vi "FourierTransform.vi"(3 "Image In":T1 {"Dialogs" format="%.0b"}) -> (0 "Complex FT":cdb[][](array[numeric]) format="%.2f", 1 "Image Out":T1 {"Dialogs" format="%.0b"})   [LabVIEW 2024]
doc: "This VI calculates the DFT (or FFT) of the image and returns the 2D complex array and puts the magnitude (log scaled) in the image area. It only works on greyscale images."
uses:
  <userlib>/ImageProcessing/QTLIB_2595_LV86/QT_Image.ctl
panel:
  # "This VI calculates the DFT (or FFT) of the image and\nreturns the 2D complex array and puts the magnitude \n(log scaled) in the image area.  It only works on greyscale images."
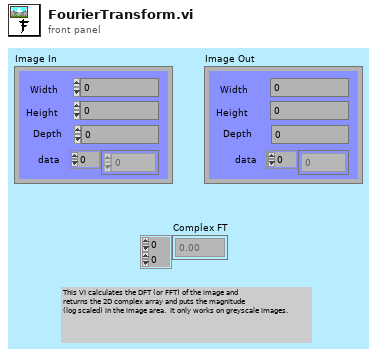
[diagram p1: front panel]
types:
  T1 = typedef "QT_Image.ctl" = cluster{"Width":i32, "Height":i32, "Depth":i32, "data":u8[], "Compressed data":u8[], "Color table":u32[], "Duration":i32, "Options":i32, "Timestamp":i32, "ID":i32, "Reserved":i32, "Dialogs":u32}
  T2 = enum16{"Same depth", "8 bit only", "1 image,8bit"}
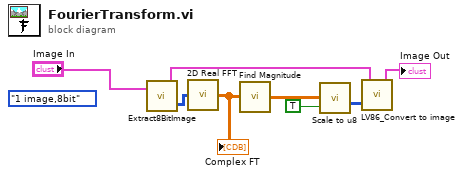
[diagram p0: block diagram]
diagram:
  (unwired) T2."1 image,8bit" ("Task")
  n1 = call <userlib>:"Extract8BitImage.vi"("Image in"="Image In") -> ("Intensity Graph"=w6:u8[][], "Image out"=w7:T1)  [unwired: 1 in]
  n2 = call <userlib>:"2D Real FFT.vi"("X"=w6) -> ("FFT {X}"=w4:cdb[][])
  "Complex FT" <- w4
  n3 = call <userlib>:"Find Magnitude.vi"("FFT {X}"=w4) -> ("Magnitude"=w3:dbl[][])
  n4 = call <userlib>:"Scale to u8.vi"("Log scaling?"=TRUE, "Intensity Graph"=w3) -> ("X"=w5:u8[][])
  n5 = call <userlib>:"LV86_Convert to image.vi"("Intensity Graph"=w5, "Image In"=w7) -> ("Image Out"=→"Image Out":T1)  [unwired: 1 in]
